vi "Read rotPA.vi"(8 "error in (no error)":errorcluster, 11 "Rotator in":refnum<class "Rotator.lvclass">) -> (0 "error out":errorcluster, 2 "rotPA":dbl[unit] min=0.0 max=6.283185307179586, 3 "Rotator out":refnum<class "Rotator.lvclass">)   [LabVIEW 2014, in "TCSDataDefinitions.lvlib" / "TCSCommand.lvlib" / "TargetConfiguration.lvlib" / "Rotator.lvclass"]
uses:
  Rotator.lvclass
  Rotator.lvclass/Rotator.ctl
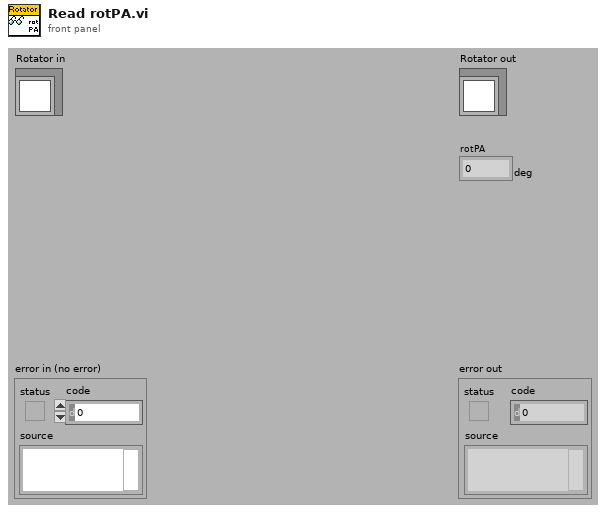
[diagram p1: front panel]
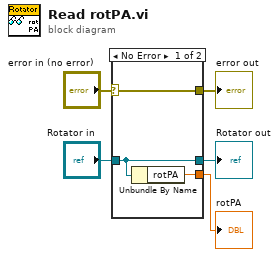
[diagram p0: block diagram]
diagram:
  n1 = case shown="No Error" "error in (no error)" {
    selector: "error in (no error)" -> [w8 w9]
    tunnel: [w8 w9] -> w4
    tunnel: [w7 w10] -> w2
    tunnel: "Rotator in" -> [w7 w10]
    tunnel: [w6 _] -> w1
    frame No Error {
      n2 = Unbundle By Name(w7) -> ("rotPA"=w6:dbl[unit])
    }
    frame Error {
    }
  }
  "error out" <- w4
  "Rotator out" <- w2
  "rotPA" <- w1
